vi "Load Plugin.vi"(8 "error in (no error)":errorcluster, 10 "Plugin":string) -> (0 "error out":errorcluster, 2 "Plugin":refnum<class "Plugin.lvclass">)   [LabVIEW 2020, in "Plugin Loader.lvclass"]
uses:
  Plugin Loader.lvclass
  Framework/Plugin/Plugin.lvclass
  Plugin Loader.lvclass/Plugin Loader.ctl
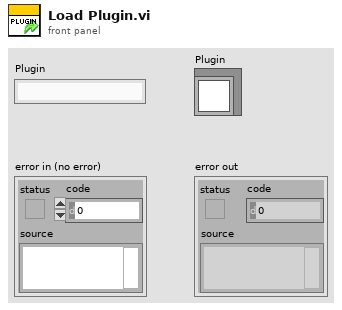
[diagram p1: front panel]
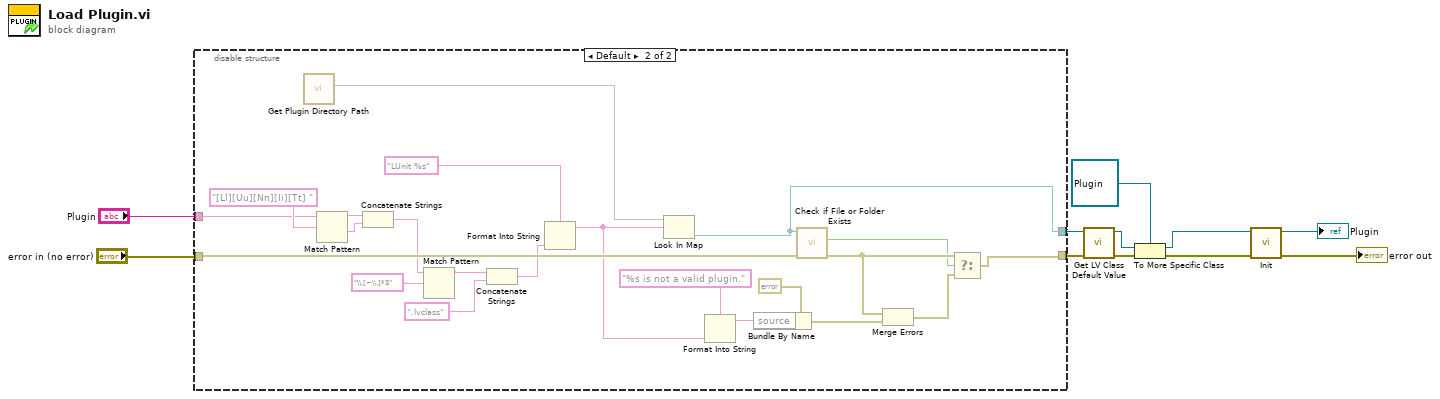
[diagram p0: block diagram]
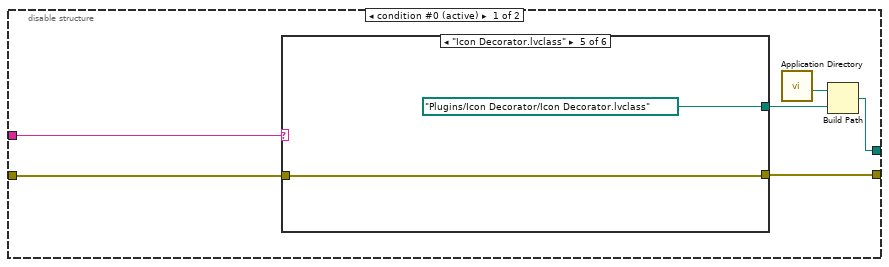
[diagram p2: hidden frame]
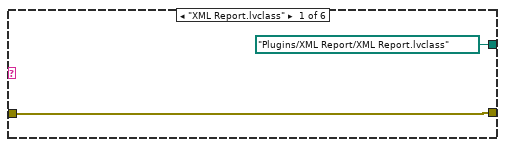
[diagram p3: hidden frame]
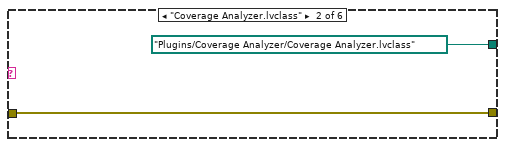
[diagram p4: hidden frame]
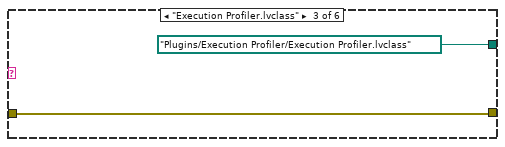
[diagram p5: hidden frame]
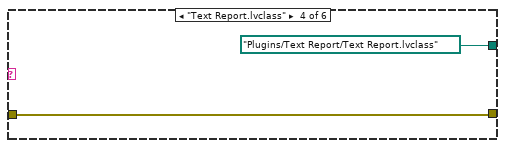
[diagram p6: hidden frame]
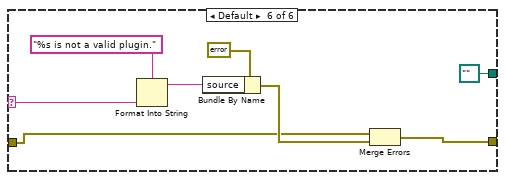
[diagram p7: hidden frame]
diagram:
  n1 = disable-structure shown="Default" {
    disable-tunnel: "Plugin" -> [w17 w44]
    disable-tunnel: "error in (no error)" -> [w16 w56]
    disable-tunnel: [w15 w50] -> w6
    disable-tunnel: [w12 w42] -> w2
    frame condition #0 (active) {
      n2 = case shown="\"Icon Decorator.lvclass\"" w17 {
        selector: w17 -> [_ _ _ _ _ w31]
        tunnel: [w19 w21 w23 w25 w27 w29] -> w15
        tunnel: w16 -> [w19 w21 w23 w25 w27 w28]
        tunnel: [path "Plugins/XML Report/XML Report.lvclass" ("name or relative path") path "Plugins/Coverage Analyzer/Coverage Analyzer.lvclass" ("Relative Path from 1 to 2") path "Plugins/Execution Profiler/Execution Profiler.lvclass" ("Relative Path from 1 to 2") path "Plugins/Text Report/Text Report.lvclass" ("Relative Path from 1 to 2") path "Plugins/Icon Decorator/Icon Decorator.lvclass" ("name or relative path") path "" ("name or relative path")] -> w13
        frame "XML Report.lvclass" {
        }
        frame "Coverage Analyzer.lvclass" {
        }
        frame "Execution Profiler.lvclass" {
        }
        frame "Text Report.lvclass" {
        }
        frame "Icon Decorator.lvclass" {
        }
        frame Default {
          n3 = Format Into String(format string="%s is not a valid plugin.", w31) -> (resulting string=w32:string)  [unwired: 2 in, 1 out]
          n4 = Bundle By Name(cluster=errorcluster {"status"=TRUE, "code"=7, "source"=""} ("error constant"), "source"=w32) -> (w34:errorcluster)
          n5 = Merge Errors(w28, w34) -> (w29:errorcluster)
        }
      }
      n6 = call <vilib>:"Application Directory.vi"() -> ("Application Directory"=w14:path)
      n7 = Build Path(base path=w14, name or relative path=w13) -> (appended path=w12:path)
    }
    frame condition #1 {
      n8 = call "Get Plugin Directory Path.vi"() -> ("Plugin map"=w43:map{string, path})  [unwired: 10 in, 1 out]
      n9 = Match Pattern(string=w44, regular expression="[Ll][Uu][Nn][Ii][Tt] ") -> (before substring=w46:string, after substring=w47:string)  [unwired: 1 in, 2 out]
      n10 = Concatenate Strings(w46, w47) -> (w38:string)
      n11 = Match Pattern(string=w38, regular expression="\\.[~\\.]*$") -> (before substring=w40:string)  [unwired: 1 in, 3 out]
      n12 = Concatenate Strings(w40, ".lvclass" ("string")) -> (w37:string)
      n13 = Format Into String(format string="LUnit %s" ("Relative Path from 1 to 2"), w37) -> (resulting string=w36:string)  [unwired: 2 in, 1 out]
      n14 = Look In Map(map=w43, key=w36) -> (value=w42:path)  [unwired: 1 in, 1 out]
      n15 = Format Into String(format string="%s is not a valid plugin.", w36) -> (resulting string=w54:string)  [unwired: 2 in, 1 out]
      n16 = Bundle By Name(cluster=errorcluster {"status"=TRUE, "code"=7, "source"=""} ("error constant"), "source"=w54) -> (w55:errorcluster)
      n17 = call <vilib>:"Check if File or Folder Exists.vi"("error in (no error)"=w56, "path"=w42) -> ("error out"=w51:errorcluster, "file or folder exists?"=w49:bool)  [unwired: 7 in, 1 out]
      n18 = Merge Errors(w51, w55) -> (w48:errorcluster)
      n19 = Select(t=w51, s=w49, f=w48) -> (s? t:f=w50:errorcluster)
    }
  }
  n20 = call <vilib>:"Get LV Class Default Value.vi"("error in (no error)"=w6, "class path"=w2) -> ("error out"=w7:errorcluster, "object"=w8:refnum<class>)  [unwired: 8 in]
  n21 = To More Specific Class(target class=refnum<class "Plugin.lvclass"> refnum ("Plugin in"), reference=w8, error in=w7) -> (specific class reference=w4:refnum<class "Plugin.lvclass">, error out=w5:errorcluster)
  n22 = call-dynamic "Init.vi"("error in (no error)"=w5, "Plugin in"=w4) -> ("error out"=→"error out":errorcluster, "Plugin out"=→"Plugin":refnum<class "Plugin.lvclass">)  [unwired: 8 in]
